vi "Inst.RP100.setLevel.vi"(8 "error in (no error)":errorcluster, 10 "Variant":variant, 11 "Inst.RP100 out":refnum<class "Inst.RP100.lvclass">) -> (0 "error out":errorcluster, 3 "Inst.RP100 out":refnum<class "Inst.RP100.lvclass">)   [LabVIEW 2019, in "Inst.RP100.lvclass"]
uses:
  Inst.RP100.lvclass
  Typedefs/Output State--Enum.ctl
  Typedefs/setLevel--Cluster.ctl
  Typedefs/Output Channel--Enum.ctl
  Inst.RP100.lvclass/Inst.RP100.ctl
  302788e2-8551-4c34-ba19-0fa0d320decd.vi
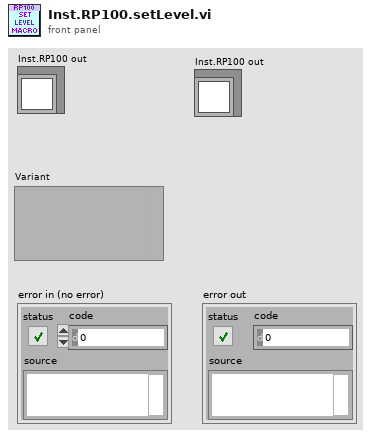
[diagram p1: front panel]
types:
  T1 = typedef "Inst.RP100.lvclass/setLevel--Cluster.ctl" = cluster{"Output Channel":T2, "Level (V)":dbl, "Slew (V/s)":dbl}
  T2 = typedef "Inst.RP100.lvclass/Output Channel--Enum.ctl" = enum16{"Output 1", "Output 2"}
  T3 = typedef "Inst.RP100.lvclass/Output State--Enum.ctl" = enum16{"Shorted", "Enabled"}
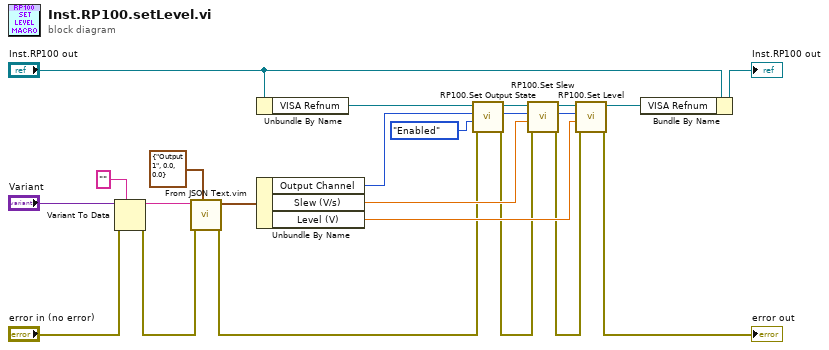
[diagram p0: block diagram]
diagram:
  n1 = Variant To Data(error in="error in (no error)", type="", Variant="Variant") -> (data=w7:string, error out=w4:errorcluster)
  n2 = call "From JSON Text.vim"("Data Type and Default Value"=T1 {"Output Channel"=enum."Output 1", "Level (V)"=0.0, "Slew (V/s)"=0.0} ("Data in"), "error in (no error)"=w4, "JSON"=w7) -> ("error out"=w2:errorcluster, "Data out"=w3:T1)  [unwired: 7 in]
  n3 = Unbundle By Name("Inst.RP100 out") -> ("VISA Refnum"=w12:refnum<visa-resource-name>)
  n4 = Unbundle By Name(w3) -> ("Output Channel"=w22:T2, "Slew (V/s)"=w21:dbl, "Level (V)"=w23:dbl)
  n5 = call "RP100.Set Output State.vi"("error in (no error)"=w2, "Output State"=Output_State--Enum."Enabled", "Output Channel"=w22, "VISA resource name"=w12) -> ("error out"=w14:errorcluster, "Output Channel"=w18:T2, "VISA Refnum out"=w17:refnum<visa-resource-name>)  [unwired: 5 in]
  n6 = call "RP100.Set Slew.vi"("error in (no error)"=w14, "Slew (V/s)"=w21, "Output Channel"=w18, "VISA resource name"=w17) -> ("error out"=w15:errorcluster, "Output Channel"=w19:T2, "VISA Refnum out"=w20:refnum<visa-resource-name>)  [unwired: 5 in]
  n7 = call "RP100.Set Level.vi"("error in (no error)"=w15, "Level (V)"=w23, "Output Channel"=w19, "VISA resource name"=w20) -> ("error out"=→"error out":errorcluster, "VISA Refnum out"=w11:refnum<visa-resource-name>)  [unwired: 5 in, 1 out]
  n8 = Bundle By Name(cluster="Inst.RP100 out", "VISA Refnum"=w11) -> (→"Inst.RP100 out":refnum<class "Inst.RP100.lvclass">)
